vi "Master_Navigator.vi"(11 "x acceleration (g)":dbl) -> (3 "Distance Out":dbl)   [LabVIEW 2017]
uses:
  <vilib>/Analysis/NI_AALPro.lvlib
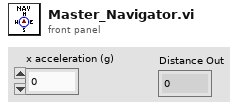
[diagram p1: front panel]
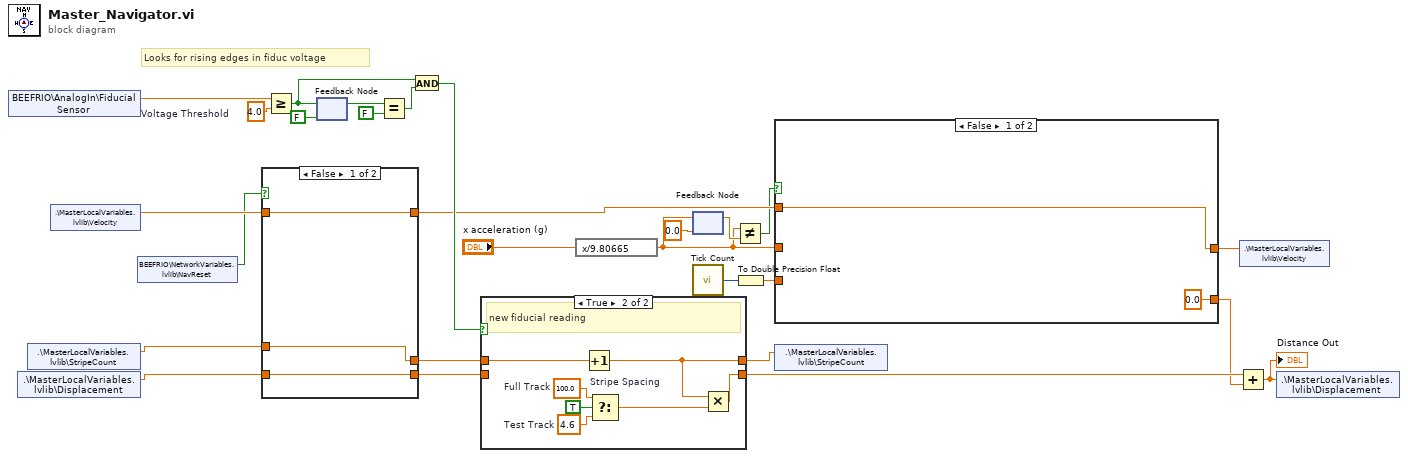
[diagram p0: block diagram]
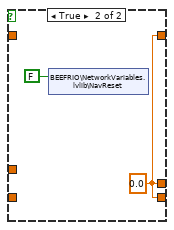
[diagram p2: hidden frame]
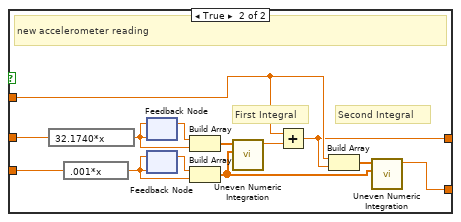
[diagram p3: hidden frame]
diagram:
  w26 = 4.0  # Voltage Threshold
  # "Looks for rising edges in fiduc voltage"
  n1 = shared-variable "BEEFRIO\\AnalogIn\\Fiducial Sensor"() -> (w27:dbl)  [unwired: 1 in, 1 out]
  n2 = shared-variable ".\\MasterLocalVariables.lvlib\\Displacement"() -> (w16:dbl)  [unwired: 1 in, 1 out]
  n3 = shared-variable ".\\MasterLocalVariables.lvlib\\StripeCount"() -> (w18:dbl)  [unwired: 1 in, 1 out]
  n4 = shared-variable ".\\MasterLocalVariables.lvlib\\Velocity"() -> (w15:dbl)  [unwired: 1 in, 1 out]
  n5 = shared-variable "BEEFRIO\\NetworkVariables.lvlib\\NavReset"() -> (w1:bool)  [unwired: 1 in, 1 out]
  n6 = case shown="False" w1 {
    tunnel: w18 -> [w30 _]
    tunnel: [w30 w32] -> w19
    tunnel: [w29 w32] -> w5
    tunnel: w16 -> [w29 _]
    tunnel: w15 -> [w28 _]
    tunnel: [w28 w32] -> w17
    frame False {
    }
    frame True {
      w32 = 0.0
      n7 = shared-variable "BEEFRIO\\NetworkVariables.lvlib\\NavReset"(FALSE ("NavReset")) -> ()  [unwired: 1 in, 1 out]
    }
  }
  n8 = Greater Or Equal?(x=w27, y=w26) -> (x >= y?=w23:bool)
  n9 = feedback-in #1(w23) -> ()
  n10 = feedback #1(FALSE) -> (w21:bool)
  n11 = Equal?(x=w21, y=FALSE) -> (x = y?=w22:bool)
  n12 = And(x=w23, y=w22) -> (x .and. y?=w20:bool)
  n13 = case shown="True" w20 {
    tunnel: [w34 w39] -> w8
    tunnel: w19 -> [w34 w41]
    tunnel: [w33 w40] -> w3
    tunnel: w5 -> [w33 _]
    frame False {
    }
    frame True {
      w38 = 4.6  # Test Track
      w37 = 100.0  # Full Track
      # "new fiducial reading"
      n14 = Increment(x=w41) -> (x+1=w39:dbl)
      n15 = Select "Stripe Spacing"(t=w37, s=TRUE, f=w38) -> (s? t:f=w36:dbl)
      n16 = Multiply(x=w39, y=w36) -> (x*y=w40:dbl)
    }
  }
  n17 = expression code="x/9.80665"("x acceleration (g)") -> (w7:dbl)
  n18 = feedback-in #2(w7) -> ()
  n19 = feedback #2(0.0 ("x acceleration (g)")) -> (w10:dbl)
  n20 = call "Tick Count"() -> ("Tick Count(mSec)"=w12:u32)
  n21 = Not Equal?(x=w7, y=w10) -> (x != y?=w9:bool)
  n22 = To Double Precision Float(number=w12) -> (double precision float=w13:dbl)
  n23 = case shown="False" w9 {
    tunnel: w17 -> [w43 w48]
    tunnel: [w43 w47] -> w14
    tunnel: w13 -> [_ w46]
    tunnel: w7 -> [_ w45]
    tunnel: [0.0 ("result") w44] -> w2
    frame False {
    }
    frame True {
      # "Second Integral"
      # "First Integral"
      # "new accelerometer reading"
      n24 = expression code="32.1740*x"(w45) -> (w54:dbl)
      n25 = expression code=".001*x"(w46) -> (w55:dbl)
      n26 = feedback #3(w54) -> (w53:dbl)
      n27 = feedback-in #3(w54) -> ()
      n28 = feedback #4(w55) -> (w49:dbl)
      n29 = feedback-in #4(w55) -> ()
      n30 = Build Array(w53, w54) -> (w50:dbl[])
      n31 = Build Array(w49, w55) -> (w52:dbl[])
      n32 = call <vilib>:"Uneven Numeric Integration.vi"("T"=w52, "X"=w50) -> ("result"=w56:dbl)  [unwired: 8 in, 1 out]
      n33 = Add(x=w48, y=w56) -> (x+y=w47:dbl)
      n34 = Build Array(w48, w47) -> (w51:dbl[])
      n35 = call <vilib>:"Uneven Numeric Integration.vi"("T"=w52, "X"=w51) -> ("result"=w44:dbl)  [unwired: 8 in, 1 out]
    }
  }
  n36 = shared-variable ".\\MasterLocalVariables.lvlib\\StripeCount"(w8) -> ()  [unwired: 1 in, 1 out]
  n37 = Add(x=w3, y=w2) -> (x+y=w4:dbl)
  "Distance Out" <- w4
  n38 = shared-variable ".\\MasterLocalVariables.lvlib\\Velocity"(w14) -> ()  [unwired: 1 in, 1 out]
  n39 = shared-variable ".\\MasterLocalVariables.lvlib\\Displacement"(w4) -> ()  [unwired: 1 in, 1 out]
